vi "subviTimingTest.vi"(9 "index":i32, 11 "array":u32[](array[numeric])) -> (3 "output array":u32[](array[numeric]))   [LabVIEW 2010]
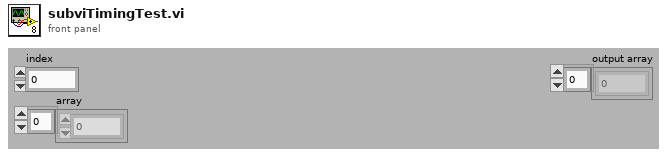
[diagram p1: front panel]
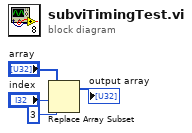
[diagram p0: block diagram]
diagram:
  n1 = Replace Array Subset(array="array", new element=u32 3 ("new element/subarray"), index="index") -> (→"output array":u32[])
